vi "Initialize Network Engine.vi"(8 "error in (no error)":errorcluster, 10 "Parameters":T3 {"Config"."Industrial Settings"."Write Refs"."Data Reference" format="%.0x"; "Config"."Industrial Settings"."Read Refs"."Data Reference" format="%.0x"; "Config"."PID Settings"."Read Refs"."Data Reference" format="%.0x"; "Config"."PID Settings"."Write Refs"."Data Reference" format="%.0x"}, 11 "Process":refnum<class "Process.lvclass">) -> (0 "error out":errorcluster, 2 "Start":bool, 3 "State Variables":T1)   [LabVIEW 2015, in "Control Addon Engine.lvlib"]
uses:
  Control Addon Engine.lvlib
  Types/RT Configuration.ctl
  Shared/Types/Gain Schedule.ctl
  Shared/Types/Compiled Settings.ctl
  Shared/Types/Compiled PID Settings.ctl
  <vilib>/NI Veristand/Custom Device API/Block Data Reference.ctl
  <vilib>/NI Veristand/Custom Device API/Data Reference.ctl
  Shared/Types/Compiled Industrial Settings.ctl
  Shared/Types/Compiled Industrial Parameters.ctl
  Types/Network Engine State Variables.ctl
  <vilib>/NI/NI VeriStand Inline Async API/_VS Inline Async API/Process/Process.lvclass
  <vilib>/NI/STM/Connection Manager/TCP/Advanced/TCP Connection Manager Reference.ctl
  <vilib>/NI/STM/Connection Manager/TCP/Advanced/TCP Connection Manager State Variables.ctl
  <vilib>/NI/STM/TCP/TCP Connection Info.ctl
  <vilib>/NI/STM/SubVIs/MetaDataElement.ctl
  <vilib>/NI/STM/Connection Manager/TCP/TCP Connection Properties.ctl
  <vilib>/NI/NI VeriStand Inline Async API/_VS Inline Async API/Process/Process.lvclass/Process.ctl
  <vilib>/NI/NI VeriStand Inline Async API/_VS Inline Async API/Error Handling Process/SubVIs/Error.ConvertArray.vi
  <vilib>/NI/STM/NI STM.lvlib
  Shared/Control Addon Shared.lvlib
  <vilib>/NI VeriStand/Custom Device API/Custom Device API.lvlib
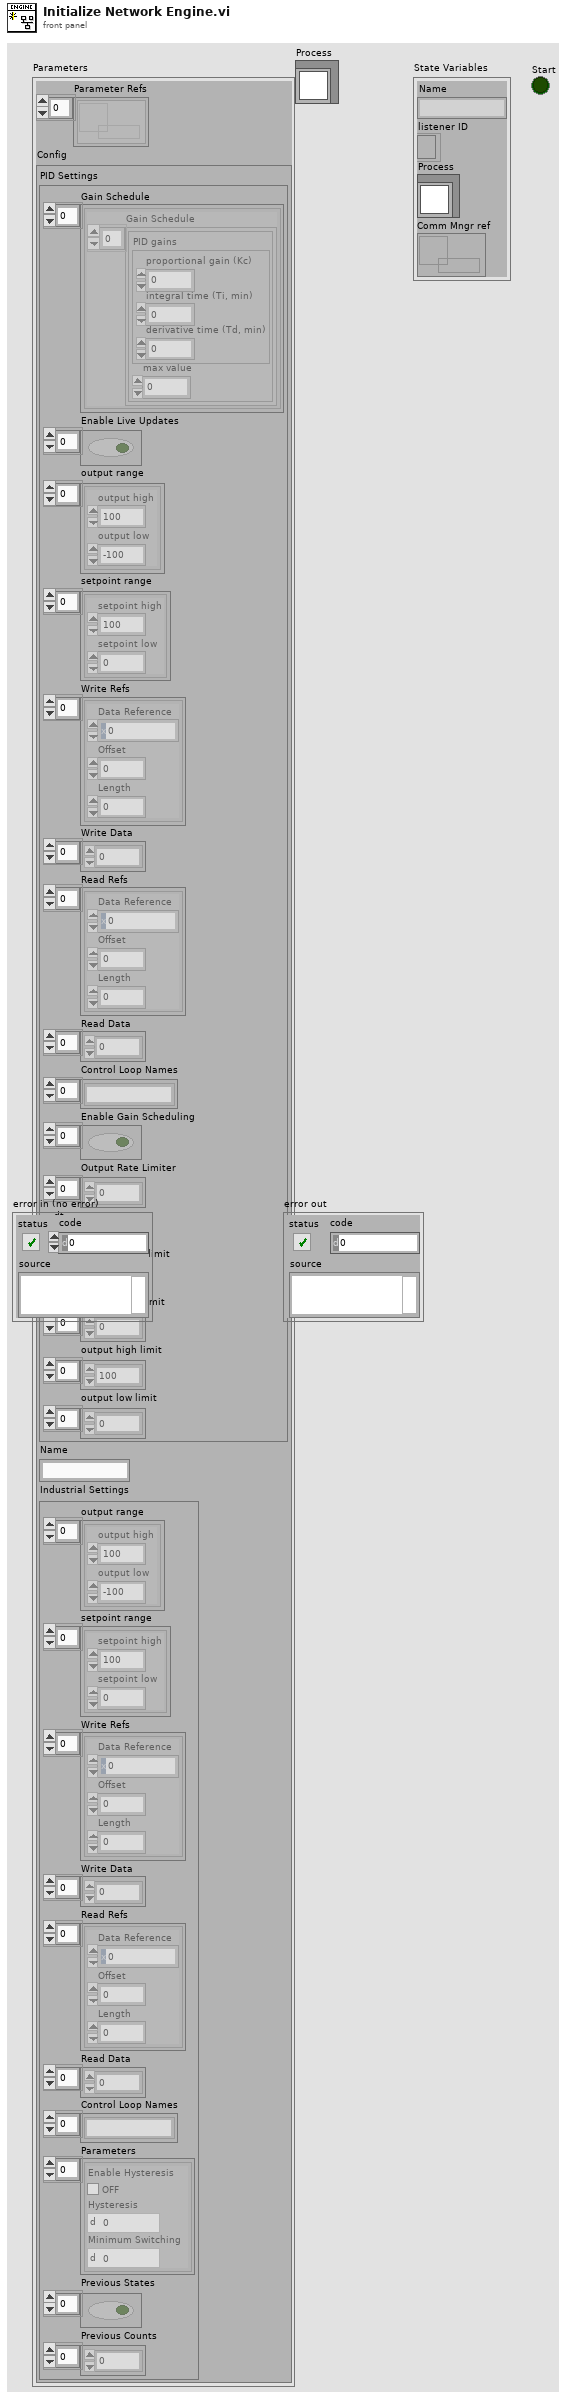
[diagram p1: front panel]
types:
  T1 = typedef "Control Addon Engine.lvlib/Network Engine State Variables.ctl" = cluster{"Name":string, "listener ID":refnum<k5>, "Process":refnum<class "Process.lvclass">, "Comm Mngr ref":T2}
  T2 = typedef "TCP Connection Manager Reference.ctl" = refnum<data-value>
  T3 = typedef "Control Addon Engine.lvlib/RT Configuration.ctl" = cluster{"Parameter Refs":refnum<data-value>[], "Config":T4}
  T4 = typedef "Control Addon Shared.lvlib/Compiled Settings.ctl" = cluster{"PID Settings":T5, "Name":string, "Industrial Settings":T9}
  T5 = typedef "Control Addon Shared.lvlib/Compiled PID Settings.ctl" = cluster{"Gain Schedule":T6[], "Enable Live Updates":bool[], "output range":cluster{"output high":dbl, "output low":dbl}[], "setpoint range":cluster{"setpoint high":dbl, "setpoint low":dbl}[], "Write Refs":T7[], "Write Data":dbl[], "Read Refs":T7[], "Read Data":dbl[], "Control Loop Names":string[], "Enable Gain Scheduling":bool[], "Output Rate Limiter":dbl[], "dt":dbl, "setpoint high limit":dbl[], "setpoint low limit":dbl[], "output high limit":dbl[], "output low limit":dbl[]}
  T6 = typedef "Control Addon Shared.lvlib/Gain Schedule.ctl" = cluster{"Gain Schedule":cluster{"PID gains":cluster{"proportional gain (Kc)":dbl, "integral time (Ti, min)":dbl, "derivative time (Td, min)":dbl}, "max value":dbl}[]}
  T7 = typedef "Custom Device API.lvlib/Block Data Reference.ctl" = cluster{"Data Reference":T8, "Offset":u64, "Length":u64}
  T8 = typedef "Custom Device API.lvlib/Data Reference.ctl" = i32
  T9 = typedef "Control Addon Shared.lvlib/Compiled Industrial Settings.ctl" = cluster{"output range":cluster{"output high":dbl, "output low":dbl}[], "setpoint range":cluster{"setpoint high":dbl, "setpoint low":dbl}[], "Write Refs":T7[], "Write Data":dbl[], "Read Refs":T7[], "Read Data":dbl[], "Control Loop Names":string[], "Parameters":T10[], "Previous States":bool[], "Previous Counts":u64[]}
  T10 = typedef "Control Addon Shared.lvlib/Compiled Industrial Parameters.ctl" = cluster{"Enable Hysteresis":bool, "Hysteresis":dbl, "Minimum Switching":u64}
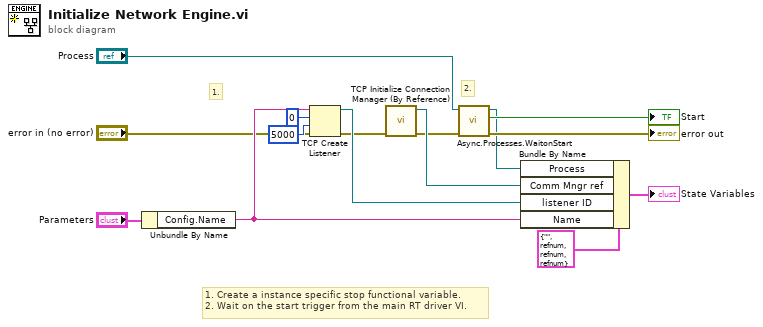
[diagram p0: block diagram]
diagram:
  # "1. Create a instance specific stop functional variable.\n2. Wait on the start trigger from the main RT driver VI."
  # "2."
  # "1."
  n1 = Unbundle By Name("Parameters") -> ("Config.Name"=w9:string)
  n2 = TCP Create Listener(8:"error in (no error)", 9:5000 ("timeout ms (25000)"), 10:u16 0 ("port"), 11:w9) -> (0:w8:errorcluster, 3:w11:refnum<k5>)  [unwired: 1 in, 1 out]
  n3 = call <vilib>:"TCP Initialize Connection Manager (By Reference).vi"("error in (no error)"=w8) -> ("error out"=w6:errorcluster, "connection manager ref out"=w10:T2)  [unwired: 9 in]
  n4 = call <vilib>:"Async.Processes.WaitonStart.vi"("error in (no error)"=w6, "Process"="Process") -> ("error out"=→"error out":errorcluster, "Execute"=→"Start":bool, "Process out"=w2:refnum<class "Process.lvclass">)  [unwired: 7 in]
  n5 = Bundle By Name(cluster=T1 {"Name"="", "listener ID"=refnum, "Process"=refnum, "Comm Mngr ref"=refnum} ("State Variables"), "Process"=w2, "Comm Mngr ref"=w10, "listener ID"=w11, "Name"=w9) -> (→"State Variables":T1)
